vi "Shooter Controller.vi"(0 "error in (no error)":errorcluster) -> ()   [LabVIEW 2011]
uses:
  Shooter Global.vi
  <vilib>/addons/control/pid/pid.llb/PID (DBL).vi
  <vilib>/addons/control/pid/NI_PID_pid.lvlib
panel:
  out "Shooter Error":errorcluster
  out "Motor Output":dbl
  out "Current Shooter Mode Being Executed":T1(ring)
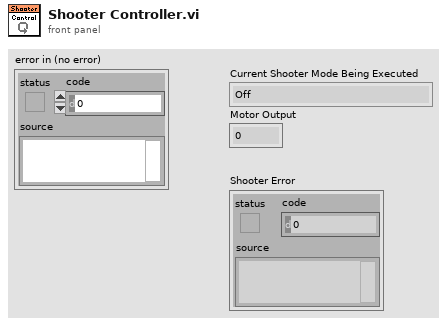
[diagram p1: front panel]
types:
  T1 = enum16{"Off", "Open Loop Control", "Closed Loop", "Top Spin", "Wait for Spindown"}
  T2 = enum16{"Off", "Open Loop Control", "Closed Loop Control", "Top Spin"}
  T3 = typedef "WPI_MotorControlDeviceRef.ctl" = cluster{"DeviceStatus":errorcluster, "Type":enum16{"PWM", "CAN"}, "PWM":cluster{"Digital Module":T4, "PWM Channel":T5, "DeadBand":T6}, "CAN":cluster{"Device Number":u8, "Control Mode":T7, "Semaphore":T8, "Max Vout":dbl}, "Invert":bool, "TransformRef":T9, "InvTransformRef":T9}
  T4 = typedef "FPGA_TypedefDigitalModule.ctl" = enum16{"Digital Module 1", "Digital Module 2"}
  T5 = typedef "FPGA_DIOPWMChannel.ctl" = enum8{"PWM 1", "PWM 2", "PWM 3", "PWM 4", "PWM 5", "PWM 6", "PWM 7", "PWM 8", "PWM 9", "PWM 10", "Invalid"}
  T6 = typedef "WPI_PWMDeadband.ctl" = cluster{"Name":string, "maxPositivePwm":i32, "minPositivePwm":i32, "centerPwm":i32, "maxNegativePwm":i32, "minNegativePwm":i32, "angularRange":u16}
  T7 = typedef "WPI_CANJaguar_ControlMode.ctl" = enum8{"Percent VBus", "Current", "Speed", "Position", "Voltage"}
  T8 = typedef "Semaphore RefNum" = refnum<k1>
  T9 = typedef "WPI_PWMTransform_ConPane.ctl" = refnum<vi>
  T10 = typedef "WPI_CounterDevRef.ctl" = cluster{"DevStatus":errorcluster, "CntIndex":T11}
  T11 = typedef "FPGA_CounterCtrSystemIndex.ctl" = enum8{"Ctr 0", "Ctr 1", "Ctr 2", "Ctr 3", "Ctr 4", "Ctr 5", "Ctr 6", "Ctr 7", "Invalid"}
  T12 = cluster{"proportional gain (Kc)":dbl, "integral time (Ti, min)":dbl, "derivative time (Td, min)":dbl}
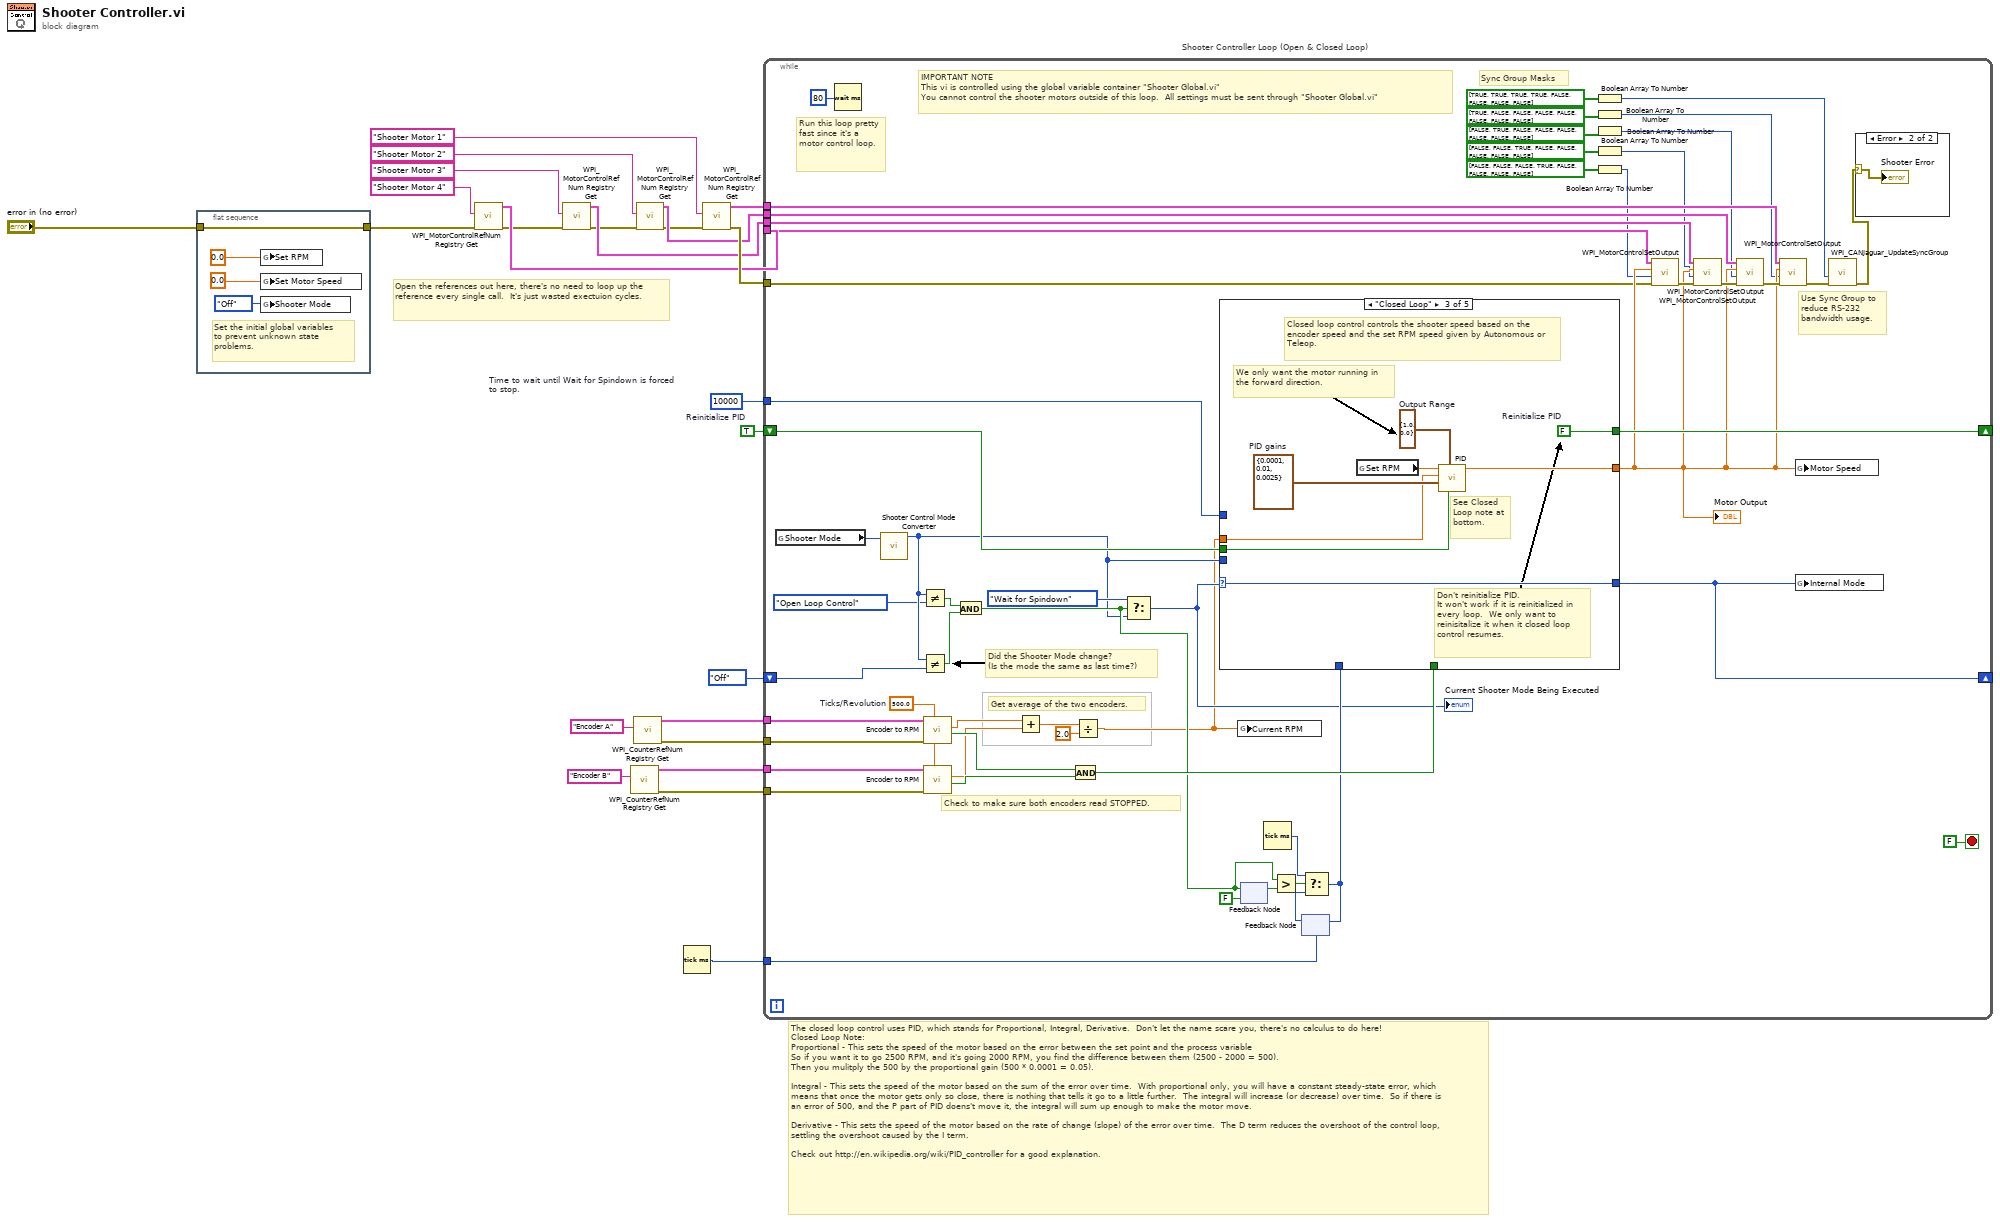
[diagram p0: block diagram]
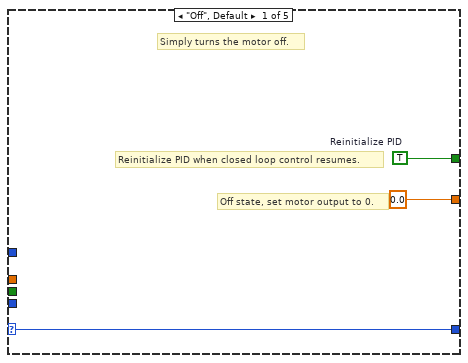
[diagram p3: hidden frame]
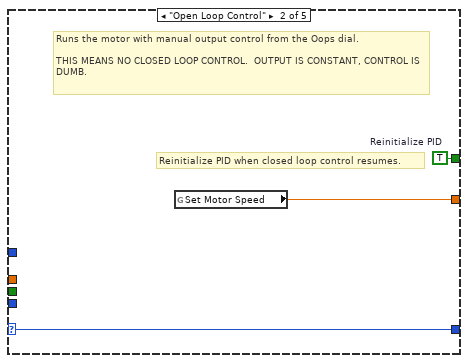
[diagram p4: hidden frame]
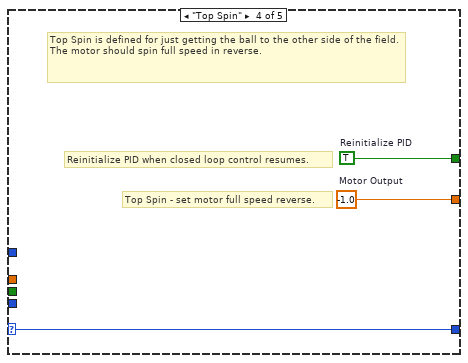
[diagram p5: hidden frame]
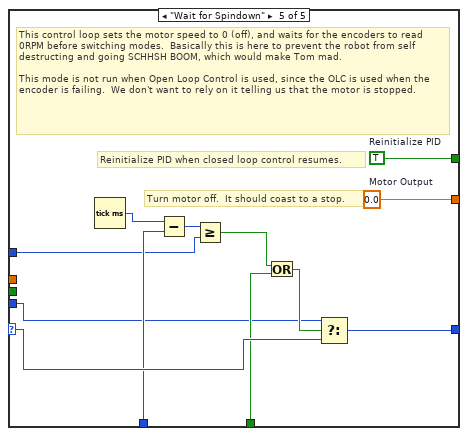
[diagram p6: hidden frame]
diagram:
  w5 = u32 10000  # Time to wait until Wait for Spindown is forced to stop.
  w18 = TRUE  # Reinitialize PID
  # "The closed loop control uses PID, which stands for Proportional, Integral, Derivative.  Don't let the name scare you, there's no calculus to do here!\nClosed Loop Note:\nProportional - This sets the speed of the motor based on the error between the set point and the process variable\nSo if you want it to go 2500 RPM, and it's going 2000 RPM, you find the difference between them (2500 - 2000 = 500).\nThen you mulitply the 500 by the proportional gain (500 * 0.0001 = 0.05).\n\nIntegral - This sets the speed of the motor based on the sum of the error over time.  With proportional only, you will have a constant steady-state error, which means that once the motor gets only so close, there is nothing that tells it go to a little further.  The integral will increase (or decrease) over time.  So if there is an error of 500, and the P part of PID doens't move it, the integral will sum up enough to make the motor move.\n\nDerivative - This sets the speed of the motor based on the rate of change (slope) of the error over time.  The D term reduces the overshoot of the control loop, settling the overshoot caused by the I term.   \n\nCheck out http://en.wikipedia.org/wiki/PID_controller for a good explanation."
  # "Open the references out here, there's no need to loop up the reference every single call.  It's just wasted exectuion cycles."
  n1 = flat-sequence {
    tunnel: [w26] -> w2
    tunnel: "error in (no error)" -> [w26]
    frame #0 {
      # "Set the initial global variables to prevent unknown state problems."
      n2 = global write "Shooter Global.vi" "Set RPM"(0.0 ("Set RPM")) -> ()
      n3 = global write "Shooter Global.vi" "Set Motor Speed"(0.0 ("Set Motor Speed")) -> ()
      n4 = global write "Shooter Global.vi" "Shooter Mode"(T2."Off" ("Shooter Mode")) -> ()
    }
  }
  n5 = call <vilib>:"WPI_MotorControlRefNum Registry Get.vi"("error in (no error)"=w2, "refnum name"="Shooter Motor 4") -> ("error out"=w7:errorcluster, "MotorControlDevRef"=w13:T3)  [unwired: 8 in]
  n6 = call <vilib>:"WPI_MotorControlRefNum Registry Get.vi"("error in (no error)"=w7, "refnum name"="Shooter Motor 3") -> ("error out"=w8:errorcluster, "MotorControlDevRef"=w14:T3)  [unwired: 8 in]
  n7 = call <vilib>:"WPI_CounterRefNum Registry Get.vi"("refnum name"="Encoder B") -> ("error out"=w22:errorcluster, "CounterDevRef"=w24:T10)  [unwired: 9 in]
  n8 = call <vilib>:"WPI_CounterRefNum Registry Get.vi"("refnum name"="Encoder A") -> ("error out"=w23:errorcluster, "CounterDevRef"=w21:T10)  [unwired: 9 in]
  n9 = call <vilib>:"WPI_MotorControlRefNum Registry Get.vi"("error in (no error)"=w8, "refnum name"="Shooter Motor 2") -> ("error out"=w9:errorcluster, "MotorControlDevRef"=w15:T3)  [unwired: 8 in]
  n10 = Tick Count (ms)() -> (millisecond timer value=w4:u32)
  n11 = call <vilib>:"WPI_MotorControlRefNum Registry Get.vi"("error in (no error)"=w9, "refnum name"="Shooter Motor 1") -> ("error out"=w17:errorcluster, "MotorControlDevRef"=w16:T3)  [unwired: 8 in]
  n12 = while "Shooter Controller Loop (Open & Closed Loop)" {
    tunnel: w13 -> [w79]
    tunnel: w14 -> [w78]
    tunnel: w15 -> [w77]
    tunnel: w16 -> [w76]
    tunnel: w17 -> [w56]
    shift-right: [w31] -> _
    shift-left: T1."Off" ("t") -> [w75]
    shift-right: [w72] -> _
    shift-left: w18 -> [w73]
    tunnel: w21 -> [w46]
    tunnel: w22 -> [w43]
    tunnel: w23 -> [w45]
    tunnel: w24 -> [w44]
    tunnel: w5 -> [w53]
    tunnel: w4 -> [w37]
    stop <- FALSE stop-if-true
    w47 = 500.0  # Ticks/Revolution
    # "IMPORTANT NOTE\nThis vi is controlled using the global variable container \"Shooter Global.vi\"\nYou cannot control the shooter motors outside of this loop.  All settings must be sent through \"Shooter Global.vi\""
    # "Did the Shooter Mode change?\n(Is the mode the same as last time?)"
    # "Use Sync Group to reduce RS-232 bandwidth usage."
    # "Run this loop pretty fast since it's a motor control loop."
    # "Check to make sure both encoders read STOPPED."
    # "Get average of the two encoders."
    # "Sync Group Masks"
    n13 = global read "Shooter Global.vi" "Shooter Mode"() -> (w34:T2)
    n14 = Wait (ms)(milliseconds to wait=u32 80) -> ()  [unwired: 1 out]
    n15 = call "Shooter Control Mode Converter.vi"("Shooter Mode"=w34) -> ("Internal Control Mode"=w33:T1)  [unwired: 10 in]
    n16 = Not Equal?(x=w33, y=T1."Open Loop Control" ("t")) -> (x != y?=w52:bool)
    n17 = Not Equal?(x=w33, y=w75) -> (x != y?=w55:bool)
    n18 = call "Encoder to RPM.vi"("CounterDevRef in"=w46, "error in (no error)"=w45, "Ticks per Revolution"=w47) -> ("RPM"=w48:dbl, "Stopped?"=w51:bool)  [unwired: 4 in, 2 out]
    n19 = call "Encoder to RPM.vi"("CounterDevRef in"=w44, "error in (no error)"=w43, "Ticks per Revolution"=w47) -> ("RPM"=w49:dbl, "Stopped?"=w50:bool)  [unwired: 4 in, 2 out]
    n20 = And(x=w52, y=w55) -> (x .and. y?=w36:bool)
    n21 = Add(x=w48, y=w49) -> (x+y=w69:dbl)
    n22 = And(x=w51, y=w50) -> (x .and. y?=w68:bool)
    n23 = Divide(x=w69, y=2.0) -> (x/y=w29:dbl)
    n24 = Select(t=T1."Wait for Spindown", s=w36, f=w33) -> (s? t:f=w35:T1)
    "Current Shooter Mode Being Executed" <- w35
    n25 = global write "Shooter Global.vi" "Current RPM"(w29) -> ()
    n26 = feedback-in #1(w36) -> ()
    n27 = feedback #1(FALSE) -> (w42:bool)
    n28 = Tick Count (ms)() -> (millisecond timer value=w54:u32)
    n29 = Greater?(x=w36, y=w42) -> (0:w40:bool)
    n30 = feedback #2(w37) -> (w38:u32)
    n31 = Select(t=w54, s=w40, f=w38) -> (s? t:f=w39:u32)
    n32 = case shown="\"Closed Loop\"" w35 {
      selector: w35 -> [w87 w90 w94 w101 w112]
      tunnel: [0.0 ("output") w91 w96 w102 w114] -> w71
      tunnel: w29 -> [_ _ w95 _ _]
      tunnel: w33 -> [_ _ _ _ w104]
      tunnel: [w87 w90 w94 w101 w113] -> w31
      tunnel: w73 -> [_ _ w93 _ _]
      tunnel: [w86 w89 w92 w100 w111] -> w72
      tunnel: w68 -> [_ _ _ _ w106]
      tunnel: w39 -> [_ _ _ _ w109]
      tunnel: w53 -> [_ _ _ _ w107]
      frame "Off", Default {
        w86 = TRUE  # Reinitialize PID
        # "Simply turns the motor off."
        # "Reinitialize PID when closed loop control resumes."
        # "Off state, set motor output to 0."
      }
      frame "Open Loop Control" {
        w89 = TRUE  # Reinitialize PID
        # "Runs the motor with manual output control from the Oops dial.\n\nTHIS MEANS NO CLOSED LOOP CONTROL.  OUTPUT IS CONSTANT, CONTROL IS DUMB."
        # "Reinitialize PID when closed loop control resumes."
        n33 = global read "Shooter Global.vi" "Set Motor Speed"() -> (w91:dbl)
      }
      frame "Closed Loop" {
        w99 = T12 {"proportional gain (Kc)"=0.0001, "integral time (Ti, min)"=0.01, "derivative time (Td, min)"=0.0025}  # PID gains
        w92 = FALSE  # Reinitialize PID
        w98 = cluster{"output high":dbl, "output low":dbl} {"output high"=1.0, "output low"=0.0}  # Output Range
        # "Closed loop control controls the shooter speed based on the encoder speed and the set RPM speed given by Autonomous or Teleop."
        # "We only want the motor running in the forward direction."
        # "Don't reinitialize PID.\nIt won't work if it is reinitialized in every loop.  We only want to reinisitalize it when it closed loop control resumes."
        # "See Closed Loop note at bottom."
        n34 = global read "Shooter Global.vi" "Set RPM"() -> (w97:dbl)
        n35 = call-poly <vilib>:"PID.vi"("reinitialize? (F)"=w93, "output range"=w98, "PID gains"=w99, "process variable"=w95, "setpoint"=w97) -> ("output"=w96:dbl)  [unwired: 5 in, 1 out]
      }
      frame "Top Spin" {
        w100 = TRUE  # Reinitialize PID
        w102 = -1.0  # Motor Output
        # "Top Spin is defined for just getting the ball to the other side of the field.  The motor should spin full speed in reverse."
        # "Top Spin - set motor full speed reverse."
        # "Reinitialize PID when closed loop control resumes."
      }
      frame "Wait for Spindown" {
        w111 = TRUE  # Reinitialize PID
        w114 = 0.0  # Motor Output
        # "This control loop sets the motor speed to 0 (off), and waits for the encoders to read 0RPM before switching modes.  Basically this is here to prevent the robot from self destructing and going SCHHSH BOOM, which would make Tom mad.\n\nThis mode is not run when Open Loop Control is used, since the OLC is used when the encoder is failing.  We don't want to rely on it telling us that the motor is stopped."
        # "Turn motor off.  It should coast to a stop."
        # "Reinitialize PID when closed loop control resumes."
        n36 = Tick Count (ms)() -> (millisecond timer value=w110:u32)
        n37 = Subtract(x=w110, y=w109) -> (x-y=w108:u32)
        n38 = Greater Or Equal?(x=w108, y=w107) -> (x >= y?=w103:bool)
        n39 = Or(x=w103, y=w106) -> (x .or. y?=w105:bool)
        n40 = Select(t=w104, s=w105, f=w112) -> (s? t:f=w113:T1)
      }
    }
    "Motor Output" <- w71
    n41 = feedback-in #2(w39) -> ()
    n42 = Boolean Array To Number(Boolean array=bool[] [TRUE, TRUE, TRUE, TRUE, FALSE, FALSE, FALSE, FALSE]) -> (number=w57:u8)
    n43 = Boolean Array To Number(Boolean array=bool[] [TRUE, FALSE, FALSE, FALSE, FALSE, FALSE, FALSE, FALSE]) -> (number=w58:u8)
    n44 = Boolean Array To Number(Boolean array=bool[] [FALSE, TRUE, FALSE, FALSE, FALSE, FALSE, FALSE, FALSE]) -> (number=w59:u8)
    n45 = Boolean Array To Number(Boolean array=bool[] [FALSE, FALSE, TRUE, FALSE, FALSE, FALSE, FALSE, FALSE]) -> (number=w60:u8)
    n46 = Boolean Array To Number(Boolean array=bool[] [FALSE, FALSE, FALSE, TRUE, FALSE, FALSE, FALSE, FALSE]) -> (number=w61:u8)
    n47 = call <vilib>:"WPI_MotorControlSetOutput.vi"("error in (no error)"=w56, "Sync Group"=w61, "Output"=w71, "MotorControlDevRef"=w79) -> ("error out"=w80:errorcluster)  [unwired: 6 in, 1 out]
    n48 = call <vilib>:"WPI_MotorControlSetOutput.vi"("error in (no error)"=w80, "Sync Group"=w60, "Output"=w71, "MotorControlDevRef"=w78) -> ("error out"=w82:errorcluster)  [unwired: 6 in, 1 out]
    n49 = call <vilib>:"WPI_MotorControlSetOutput.vi"("error in (no error)"=w82, "Sync Group"=w59, "Output"=w71, "MotorControlDevRef"=w77) -> ("error out"=w81:errorcluster)  [unwired: 6 in, 1 out]
    n50 = call <vilib>:"WPI_MotorControlSetOutput.vi"("error in (no error)"=w81, "Sync Group"=w58, "Output"=w71, "MotorControlDevRef"=w76) -> ("error out"=w67:errorcluster)  [unwired: 6 in, 1 out]
    n51 = global write "Shooter Global.vi" "Motor Speed"(w71) -> ()
    n52 = global write "Shooter Global.vi" "Internal Mode"(w31) -> ()
    n53 = call <vilib>:"WPI_CANJaguar_UpdateSyncGroup.vi"("error in (no error)"=w67, "Sync Group"=w57) -> ("error out"=w30:errorcluster)  [unwired: 9 in]
    n54 = case shown="Error" w30 {
      selector: w30 -> [_ w85]
      frame No Error {
      }
      frame Error {
        "Shooter Error" <- w85
      }
    }
  }
